vi "Load FGen Waveform.vi"(8 "error in (no error)":errorcluster, 10 "Function Generator":T1, 11 "Program Data":T4={"Measurements"={"Channel 0"="Channel 0", "RMS 0"="RMS:", "Vp-p 0"="Vp-p:", "Freq 0"="Freq:", "Channel 1"="Channel 1", "RMS 1"="RMS:", "Vp-p 1"="Vp-p:", "Freq 1"="Freq:", "Cursors"="Channel 0", "C1"="Channel 0", "C2"="Channel 0", "dT"="Channel 0"}, "C1"={"Name"="", "X"=0.0, "Y"=0.0}, "C2"={"Name"="", "X"=0.0, "Y"=0.0}, "Com"={"Connection Info"={"connection ID"=refnum, "meta data"=[]}, "Connected?"=FALSE, "IP"=""}, "Continuous?"=FALSE, "Scope Data"={"AI0"=[], "AI1"=[]}, "Wave Parameters"={"Frequency (Hz)"=5.0, "Phase offset (deg)"=0.0, "Vpeak (V)"=5.0, "Offset (V)"=0.0, "Waveform"=enum."Sine", "Channel"=enum."CH0"}, "Acquire?"=FALSE, "Measure Ref"=refnum, "CH0"={"Channel"=enum."AI 0", "Enable"=FALSE, "Volts/Div"=0, "Vertical Position (Div)"=0.0}, "CH1"={"Channel"=enum."AI 0", "Enable"=FALSE, "Volts/Div"=0, "Vertical Position (Div)"=0.0}, "CH0 Params"={"V/Div"=0.0, "Units"=""}, "CH1 Params"={"V/Div"=0.0, "Units"=""}, "Time"={"Time/Div"=0.0}, "dT"=0.0, "FGen"={"Offset (V)"=0.0, "Enable Sweep"=FALSE, "Start Frequency (Hz)"=0.0, "Stop Frequency (Hz)"=0.0, "Step (Hz)"=0.0, "Step Interval (ms)"=0.0, "Current Freq (Hz)"=0.0, "Run"=FALSE}} {"Time"."Time/Div" min=0.0 max=16.0 step=1.0 scale=0.0..12.0; "CH1"."Vertical Position (Div)" min=-5.0 max=5.0 step=0.1 scale=-5.0..5.0; "CH1"."Volts/Div" min=0 max=8 step=1 scale=0.0..8.0; "CH0"."Vertical Position (Div)" min=-5.0 max=5.0 step=0.1 scale=-5.0..5.0; "CH0"."Volts/Div" min=0 max=8 step=1 scale=0.0..8.0; "Wave Parameters"."Phase offset (deg)" format="%#_6p"; "Wave Parameters"."Frequency (Hz)" format="%#_6p"}) -> (0 "error out":errorcluster, 3 "Program Data Out":T4={"Measurements"={"Channel 0"="Channel 0", "RMS 0"="RMS:", "Vp-p 0"="Vp-p:", "Freq 0"="Freq:", "Channel 1"="Channel 1", "RMS 1"="RMS:", "Vp-p 1"="Vp-p:", "Freq 1"="Freq:", "Cursors"="Channel 0", "C1"="Channel 0", "C2"="Channel 0", "dT"="Channel 0"}, "C1"={"Name"="", "X"=0.0, "Y"=0.0}, "C2"={"Name"="", "X"=0.0, "Y"=0.0}, "Com"={"Connection Info"={"connection ID"=refnum, "meta data"=[]}, "Connected?"=FALSE, "IP"=""}, "Continuous?"=FALSE, "Scope Data"={"AI0"=[], "AI1"=[]}, "Wave Parameters"={"Frequency (Hz)"=5.0, "Phase offset (deg)"=0.0, "Vpeak (V)"=5.0, "Offset (V)"=0.0, "Waveform"=enum."Sine", "Channel"=enum."CH0"}, "Acquire?"=FALSE, "Measure Ref"=refnum, "CH0"={"Channel"=enum."AI 0", "Enable"=FALSE, "Volts/Div"=0, "Vertical Position (Div)"=0.0}, "CH1"={"Channel"=enum."AI 0", "Enable"=FALSE, "Volts/Div"=0, "Vertical Position (Div)"=0.0}, "CH0 Params"={"V/Div"=0.0, "Units"=""}, "CH1 Params"={"V/Div"=0.0, "Units"=""}, "Time"={"Time/Div"=0.0}, "dT"=0.0, "FGen"={"Offset (V)"=0.0, "Enable Sweep"=FALSE, "Start Frequency (Hz)"=0.0, "Stop Frequency (Hz)"=0.0, "Step (Hz)"=0.0, "Step Interval (ms)"=0.0, "Current Freq (Hz)"=0.0, "Run"=FALSE}} {"Time"."Time/Div" min=0.0 max=16.0 step=1.0 scale=0.0..12.0; "CH1"."Vertical Position (Div)" min=-5.0 max=5.0 step=0.1 scale=-5.0..5.0; "CH1"."Volts/Div" min=0 max=8 step=1 scale=0.0..8.0; "CH0"."Vertical Position (Div)" min=-5.0 max=5.0 step=0.1 scale=-5.0..5.0; "CH0"."Volts/Div" min=0 max=8 step=1 scale=0.0..8.0; "Wave Parameters"."Phase offset (deg)" format="%#_6p"; "Wave Parameters"."Frequency (Hz)" format="%#_6p"})   [LabVIEW 2021]
uses:
  Controls/Program Data.ctl
  Controls/Measurements.ctl
  Controls/Channel Measurement String Control.ctl
  Controls/Cursor Info.ctl
  Controls/Communication Cluster.ctl
  <vilib>/NI/STM/TCP/TCP Connection Info.ctl
  <vilib>/NI/STM/SubVIs/MetaDataElement.ctl
  Communication/Scope Data.ctl
  Program Files (x86)/National Instruments/LabVIEW 2021/ProjectTemplates/Source/myRIO/Oscilloscope/myRIO v1.1/Real-Time/Controls/Wave Parameters.ctl
  Program Files (x86)/National Instruments/LabVIEW 2021/ProjectTemplates/Source/myRIO/Oscilloscope/myRIO v1.1/Real-Time/Controls/Waveform Enum.ctl
  Program Files (x86)/National Instruments/LabVIEW 2021/ProjectTemplates/Source/myRIO/Oscilloscope/myRIO v1.1/Real-Time/Controls/Channel Selector.ctl
  Controls/Channel Settings.ctl
  Controls/Analog Input Selector.ctl
  Controls/Knob.ctl
  Controls/Vertical Position.ctl
  Controls/Channel Parameters.ctl
  Controls/Time Selector.ctl
  Controls/Time Knob.ctl
  Controls/FGen Desktop Configuration.ctl
  Controls/Function Generator Control.ctl
  <vilib>/NI/STM/NI STM.lvlib
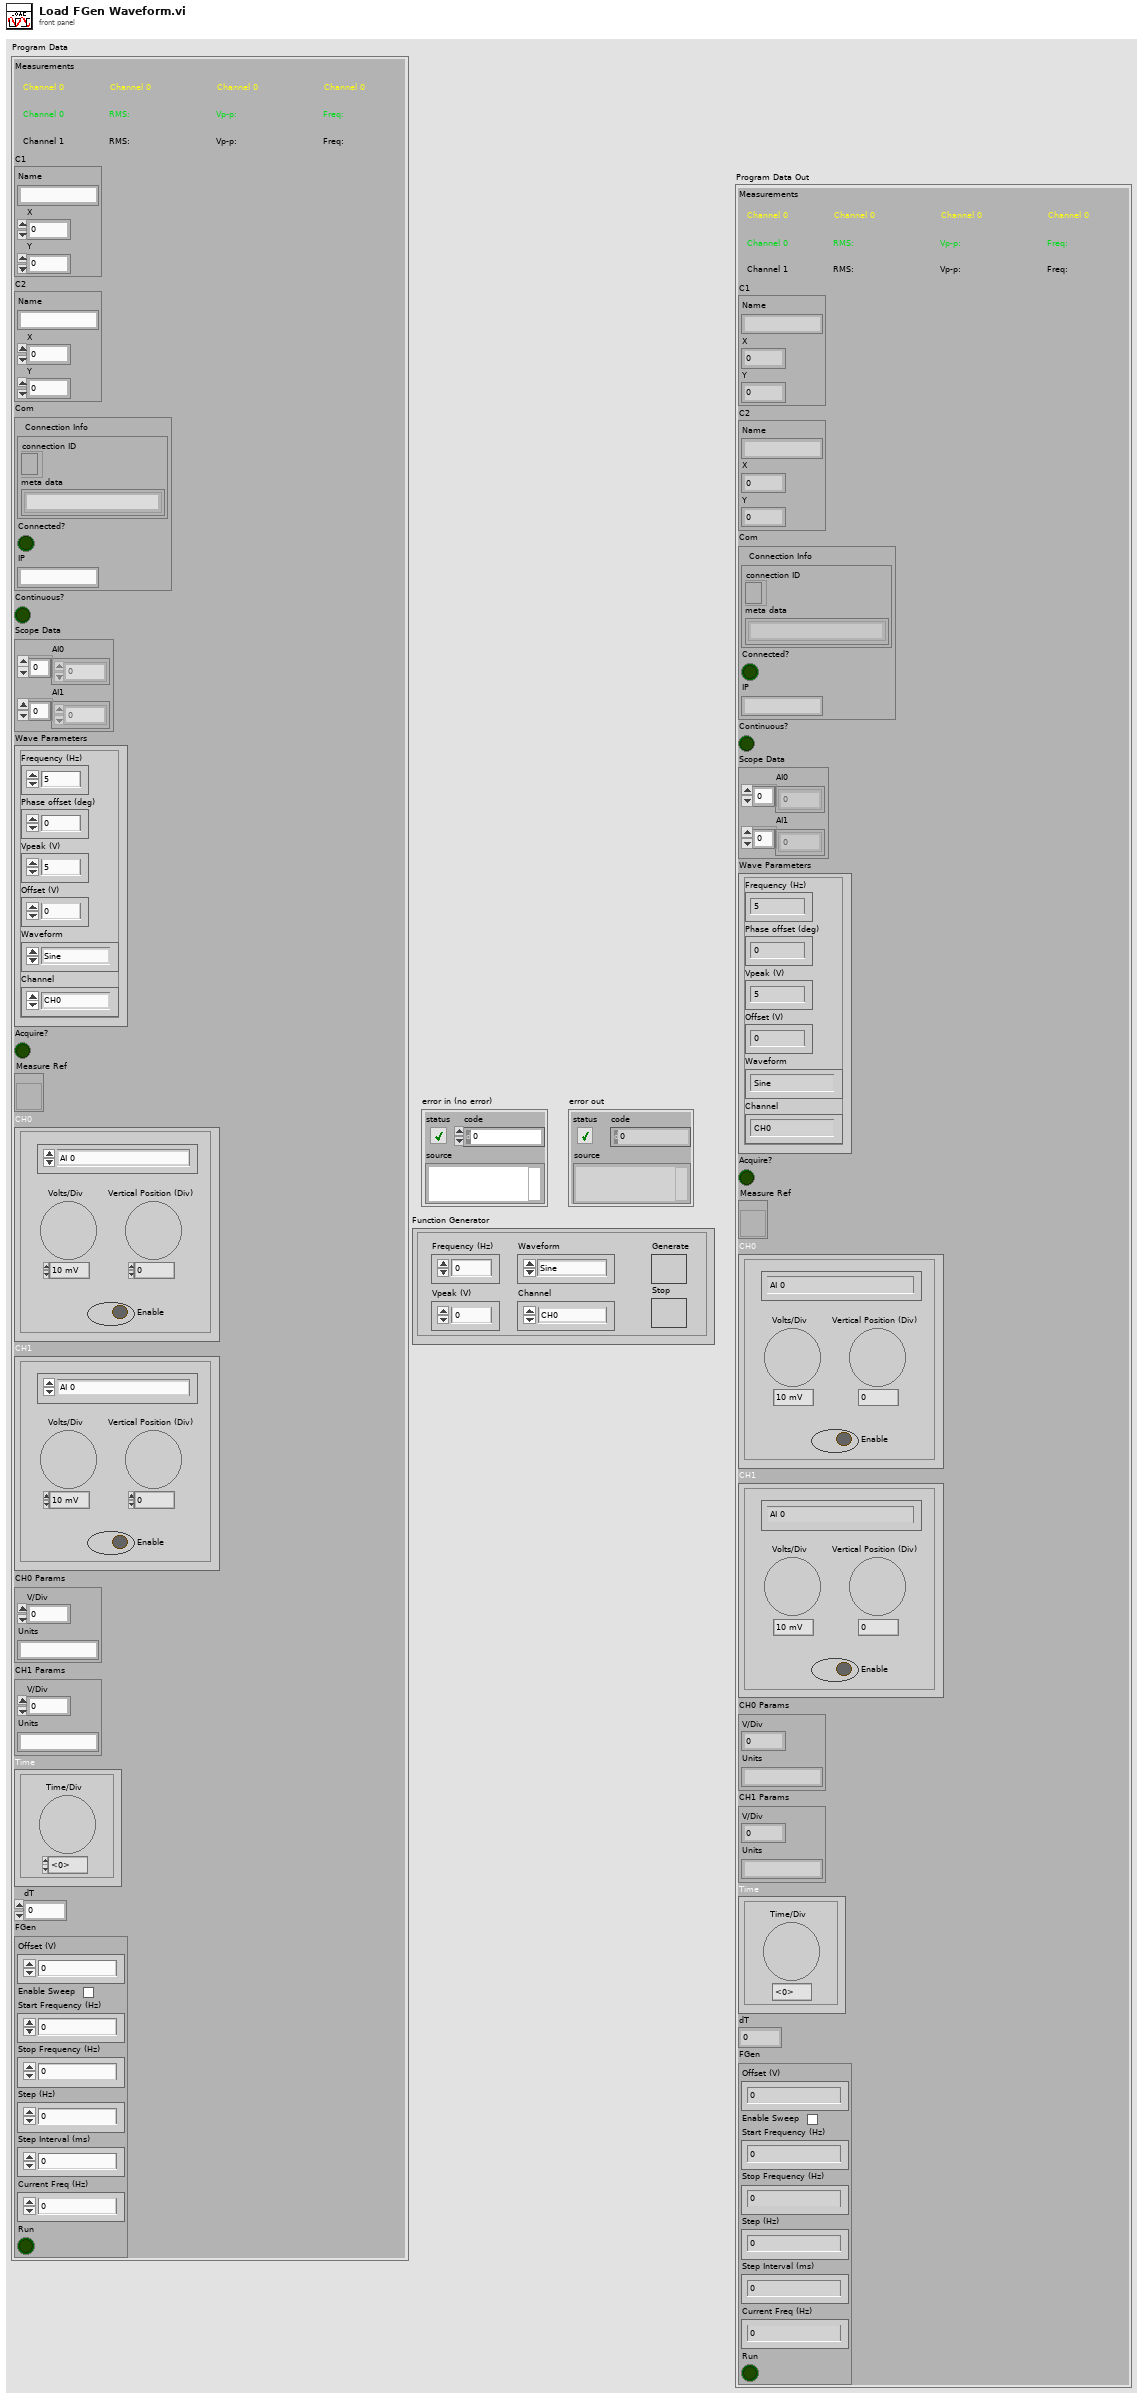
[diagram p1: front panel]
types:
  T1 = typedef "Function Generator Control.ctl" = cluster{"Frequency (Hz)":dbl, "Vpeak (V)":dbl, "Waveform":T2, "Channel":T3, "Generate":bool, "Stop":bool}
  T2 = typedef "Waveform Enum.ctl" = enum16{"Sine", "Square"}
  T3 = typedef "Channel Selector.ctl" = enum16{"CH0", "CH1"}
  T4 = typedef "Program Data.ctl" = cluster{"Measurements":T5, "C1":T7, "C2":T7, "Com":T8, "Continuous?":bool, "Scope Data":T11, "Wave Parameters":T12, "Acquire?":bool, "Measure Ref":refnum<vi>, "CH0":T13, "CH1":T13, "CH0 Params":T17, "CH1 Params":T17, "Time":T18, "dT":dbl, "FGen":T20}
  T5 = typedef "Measurements.ctl" = cluster{"Channel 0":T6, "RMS 0":T6, "Vp-p 0":T6, "Freq 0":T6, "Channel 1":T6, "RMS 1":T6, "Vp-p 1":T6, "Freq 1":T6, "Cursors":T6, "C1":T6, "C2":T6, "dT":T6}
  T6 = typedef "Channel Measurement String Control.ctl" = string
  T7 = typedef "Cursor Info.ctl" = cluster{"Name":string, "X":dbl, "Y":dbl}
  T8 = typedef "Communication Cluster.ctl" = cluster{"Connection Info":T9, "Connected?":bool, "IP":string}
  T9 = typedef "NI STM.lvlib/TCP Connection Info.ctl" = cluster{"connection ID":refnum<k5>, "meta data":T10[]}
  T10 = typedef "NI STM.lvlib/MetaDataElement.ctl" = string
  T11 = typedef "Scope Data.ctl" = cluster{"AI0":dbl[], "AI1":dbl[]}
  T12 = typedef "Wave Parameters.ctl" = cluster{"Frequency (Hz)":dbl, "Phase offset (deg)":dbl, "Vpeak (V)":dbl, "Offset (V)":dbl, "Waveform":T2, "Channel":T3}
  T13 = typedef "Channel Settings.ctl" = cluster{"Channel":T14, "Enable":bool, "Volts/Div":T15, "Vertical Position (Div)":T16}
  T14 = typedef "Analog Input Selector.ctl" = enum16{"AI 0", "AI 1"}
  T15 = typedef "Knob.ctl" = i32
  T16 = typedef "Vertical Position.ctl" = dbl
  T17 = typedef "Channel Parameters.ctl" = cluster{"V/Div":dbl, "Units":string}
  T18 = typedef "Time Selector.ctl" = cluster{"Time/Div":T19}
  T19 = typedef "Time Knob.ctl" = dbl
  T20 = typedef "FGen Desktop Configuration.ctl" = cluster{"Offset (V)":dbl, "Enable Sweep":bool, "Start Frequency (Hz)":dbl, "Stop Frequency (Hz)":dbl, "Step (Hz)":dbl, "Step Interval (ms)":dbl, "Current Freq (Hz)":dbl, "Run":bool}
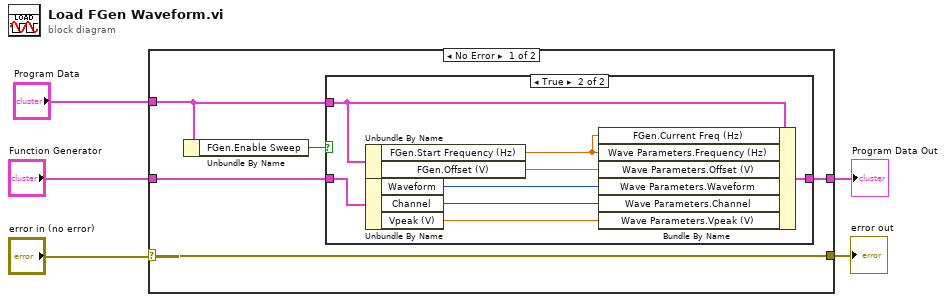
[diagram p0: block diagram]
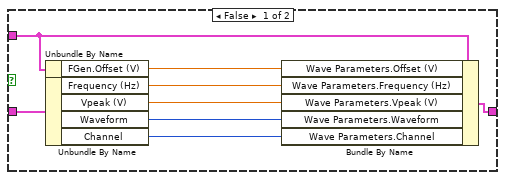
[diagram p2: hidden frame]
diagram:
  n1 = case shown="No Error" "error in (no error)" {
    selector: "error in (no error)" -> [w8 w28]
    tunnel: "Program Data" -> [w7 w27]
    tunnel: [w10 w27] -> w4
    tunnel: "Function Generator" -> [w9 _]
    tunnel: [w8 w28] -> w1
    frame No Error {
      n2 = Unbundle By Name(w7) -> ("FGen.Enable Sweep"=w6:bool)
      n3 = case shown="True" w6 {
        tunnel: [w18 w26] -> w10
        tunnel: w9 -> [w17 w23]
        tunnel: w7 -> [w12 w25]
        frame False {
          n4 = Unbundle By Name(w12) -> ("FGen.Offset (V)"=w11:dbl)
          n5 = Unbundle By Name(w17) -> ("Frequency (Hz)"=w16:dbl, "Vpeak (V)"=w15:dbl, "Waveform"=w14:T2, "Channel"=w13:T3)
          n6 = Bundle By Name(cluster=w12, "Wave Parameters.Offset (V)"=w11, "Wave Parameters.Frequency (Hz)"=w16, "Wave Parameters.Vpeak (V)"=w15, "Wave Parameters.Waveform"=w14, "Wave Parameters.Channel"=w13) -> (w18:T4)
        }
        frame True {
          n7 = Unbundle By Name(w25) -> ("FGen.Start Frequency (Hz)"=w19:dbl, "FGen.Offset (V)"=w24:dbl)
          n8 = Unbundle By Name(w23) -> ("Waveform"=w22:T2, "Channel"=w21:T3, "Vpeak (V)"=w20:dbl)
          n9 = Bundle By Name(cluster=w25, "FGen.Current Freq (Hz)"=w19, "Wave Parameters.Frequency (Hz)"=w19, "Wave Parameters.Offset (V)"=w24, "Wave Parameters.Waveform"=w22, "Wave Parameters.Channel"=w21, "Wave Parameters.Vpeak (V)"=w20) -> (w26:T4)
        }
      }
    }
    frame Error {
    }
  }
  "Program Data Out" <- w4
  "error out" <- w1
